vi "AMC e.bloxx Check Module Status.vi"(8 "error in (no error)":errorcluster, 10 "Throw LabVIEW Error (F)":bool, 11 "Module Status":i32) -> (0 "error out":errorcluster, 2 "Any Errors?":bool, 3 "Module Errors":T1[](array[typedef]) items=["EEPROM Error", "FLASH Error", "ADC Error", "Configuration Error"])   [LabVIEW 2013]
doc: "<B>AMC - Analytik & Messtechnik GmbH Chemnitz</B>\n\nLabVIEW Drivers for e.bloxx series from Gantner Instruments\n\nThis VI checks the module status specified by <B>Module Status</B>. It returns an array of defined errors. If <B>Throw LabVIEW Error</B> is true and a module error is present, <B>error out</B> receives an error 6000."
uses:
  AMC e.bloxx Module Error.ctl
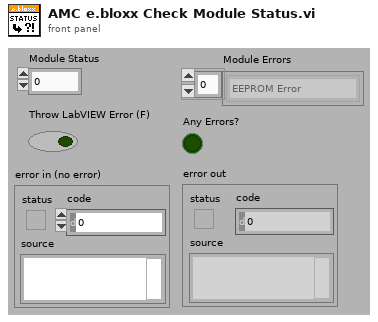
[diagram p1: front panel]
types:
  T1 = typedef "AMC e.bloxx Module Error.ctl" = i32
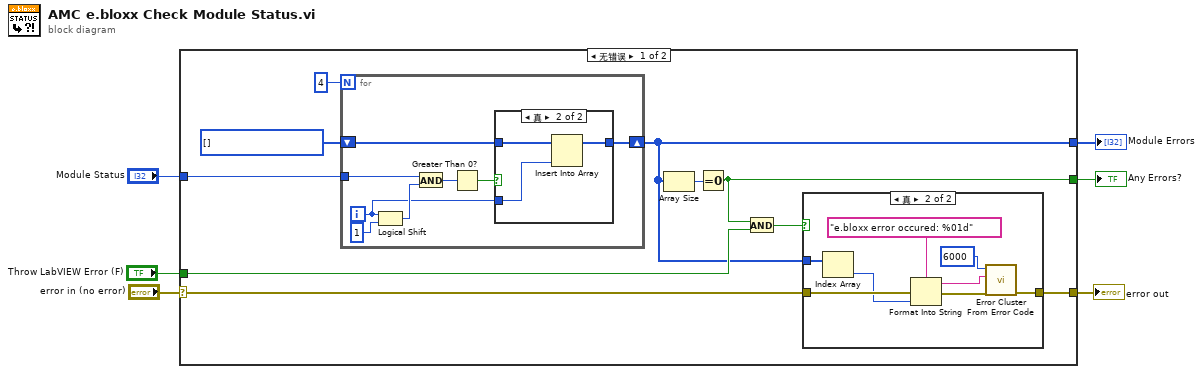
[diagram p0: block diagram]
diagram:
  n1 = case shown="无错误" "error in (no error)" {
    selector: "error in (no error)" -> [w13 w38]
    tunnel: "Module Status" -> [w15 _]
    tunnel: [w9 _] -> w4
    tunnel: [w7 _] -> w3
    tunnel: "Throw LabVIEW Error (F)" -> [w10 _]
    tunnel: [w12 w38] -> w1
    frame No Error {
      w14 = T1[] [] items=["EEPROM Error", "FLASH Error", "ADC Error", "Configuration Error"] ("Module Errors")
      n2 = for {
        N: 4 -> [_]
        tunnel: w15 -> [w32]
        shift-right: [w26] -> w9
        shift-left: w14 -> [w28]
        i -> [w27]
        n3 = Logical Shift(y=w27, x=1) -> (x << y=w31:i32)
        n4 = And(x=w32, y=w31) -> (x .and. y?=w30:i32)
        n5 = Greater Than 0?(x=w30) -> (x > 0?=w29:bool)
        n6 = case shown="真" w29 {
          tunnel: w28 -> [w34 w37]
          tunnel: w27 -> [_ w35]
          tunnel: [w34 w36] -> w26
          frame False {
          }
          frame True {
            n7 = Insert Into Array(array=w37, new element=w35) -> (w36:T1[])  [unwired: 1 in]
          }
        }
      }
      n8 = Array Size(array=w9) -> (size(s)=w8:i32)
      n9 = Equal To 0?(x=w8) -> (x = 0?=w7:bool)
      n10 = And(x=w7, y=w10) -> (x .and. y?=w11:bool)
      n11 = case shown="真" w11 {
        tunnel: w13 -> [w17 w22]
        tunnel: [w17 w25] -> w12
        tunnel: w9 -> [_ w23]
        frame False {
        }
        frame True {
          n12 = Index Array(array=w23) -> (element=w19:T1)  [unwired: 1 in]
          n13 = Format Into String(format string="e.bloxx error occured: %01d", error in=w22, w19) -> (resulting string=w18:string, error out=w21:errorcluster)  [unwired: 1 in]
          n14 = call <vilib>:"Error Cluster From Error Code.vi"("error in (no error)"=w21, "error message (\"\")"=w18, "error code (0)"=6000) -> ("error out"=w25:errorcluster)  [unwired: 6 in]
        }
      }
    }
    frame Error {
    }
  }
  "Module Errors" <- w4
  "Any Errors?" <- w3
  "error out" <- w1
